vi "BRig_Host__Loop_Consumer_RunState__typeTrial__subtypeSelResult_parse__v3.vi"(0 "input_strCmd":string) -> (3 "output_selResult":bool, 4 "output_nTrial":u16, 6 "output_sSelection":u16, 8 "output_tSelection":u16, 10 "output_iReward_or_iError":u16, 12 "output_DAB_flipLR":u16, 13 "output_trig_l2":u16, 14 "output_trig_l1":u16, 15 "output_LorR":u16)   [LabVIEW 2014]
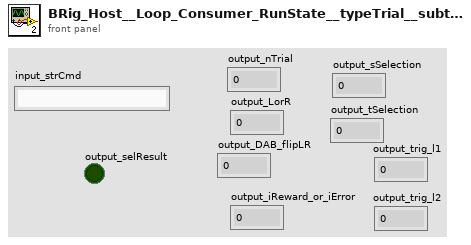
[diagram p1: front panel]
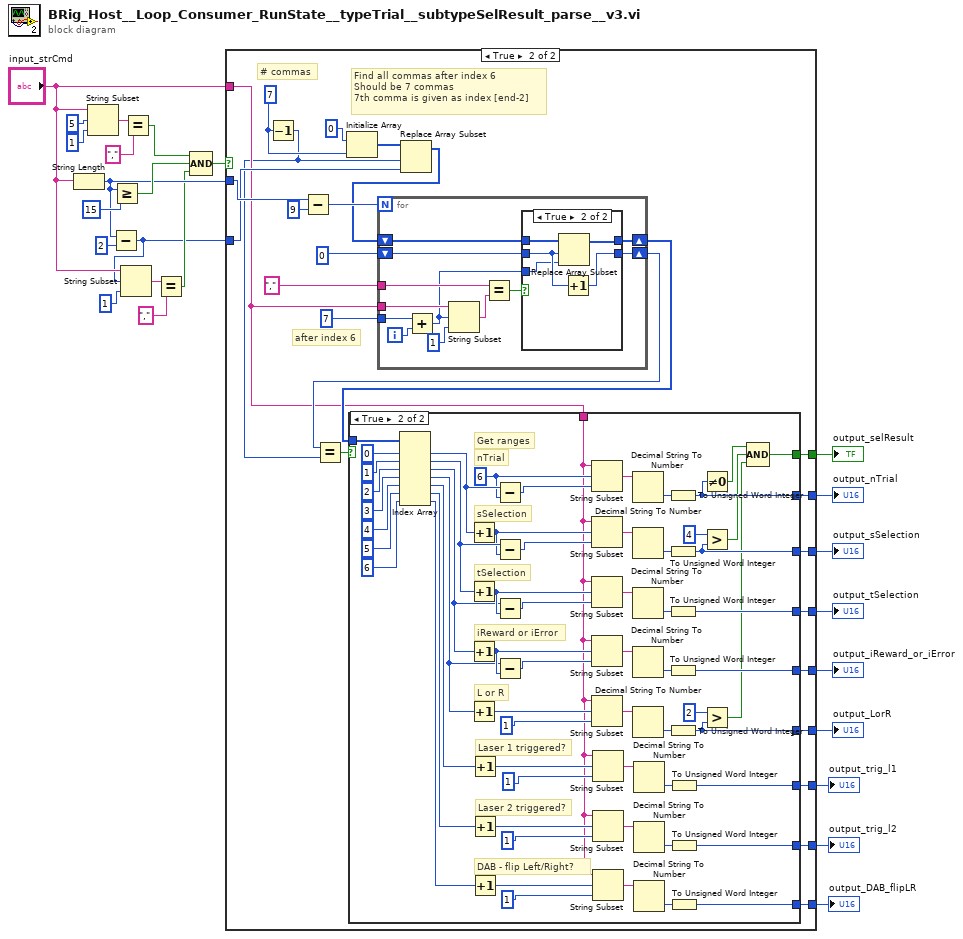
[diagram p0: block diagram]
diagram:
  n1 = String Length(string="input_strCmd") -> (length=w13:i32)
  n2 = String Subset(string="input_strCmd", offset (0)=5, length (rest)=1 ("offset (0)")) -> (substring=w23:string)
  n3 = Subtract(x=w13, y=2) -> (x-y=w10:i32)
  n4 = Greater Or Equal?(x=w13, y=15) -> (x >= y?=w20:bool)
  n5 = String Subset(string="input_strCmd", offset (0)=w10, length (rest)=1 ("offset (0)")) -> (substring=w15:string)
  n6 = Equal?(x=w23, y=",") -> (x = y?=w19:bool)
  n7 = Equal?(x=w15, y=",") -> (x = y?=w11:bool)
  n8 = Compound Arithmetic op=AND(w19, w20, w11) -> (w18:bool)
  n9 = case shown="True" w18 {
    tunnel: "input_strCmd" -> [_ w38]
    tunnel: w13 -> [_ w48]
    tunnel: w10 -> [_ w40]
    tunnel: [_ w36] -> w9
    tunnel: [_ w35] -> w8
    tunnel: [_ w34] -> w7
    tunnel: [_ w33] -> w6
    tunnel: [_ w32] -> w5
    tunnel: [_ w31] -> w4
    tunnel: [_ w28] -> w3
    tunnel: [_ w27] -> w2
    tunnel: [_ w26] -> w1
    frame False {
    }
    frame True {
      w30 = 7 ("dimension size")
      # "# commas"
      # "after index 6"
      # "Find all commas after index 6\nShould be 7 commas\n7th comma is given as index [end-2]"
      n10 = Decrement(x=w30) -> (x-1=w29:i32)
      n11 = Subtract(x=w48, y=9) -> (x-y=w47:i32)
      n12 = Initialize Array(0 ("element"), w30) -> (w42:i32[])
      n13 = Replace Array Subset(array=w42, new element=w40, index=w29) -> (w41:i32[])
      n14 = for {
        N: w47 -> [_]
        tunnel: w38 -> [w123]
        tunnel: "," ("y") -> [w121]
        tunnel: 7 ("element") -> [w119]
        shift-right: [w113] -> w43
        shift-left: 0 ("element") -> [w115]
        shift-right: [w114] -> w39
        shift-left: w41 -> [w116]
        i -> [w120]
        n15 = Add(x=w119, y=w120) -> (x+y=w117:i32)
        n16 = String Subset(string=w123, offset (0)=w117, length (rest)=1 ("offset (0)")) -> (substring=w122:string)
        n17 = Equal?(x=w121, y=w122) -> (x = y?=w118:bool)
        n18 = case shown="True" w118 {
          tunnel: w117 -> [_ w128]
          tunnel: w116 -> [w126 w131]
          tunnel: w115 -> [w125 w129]
          tunnel: [w126 w130] -> w114
          tunnel: [w125 w127] -> w113
          frame False {
          }
          frame True {
            n19 = Replace Array Subset(array=w131, new element=w128, index=w129) -> (w130:i32[])
            n20 = Increment(x=w129) -> (x+1=w127:i32)
          }
        }
      }
      n21 = Equal?(x=w43, y=w29) -> (x = y?=w37:bool)
      n22 = case shown="True" w37 {
        tunnel: w39 -> [_ w112]
        tunnel: w38 -> [_ w51]
        tunnel: [_ w81] -> w36
        tunnel: [_ w77] -> w35
        tunnel: [_ w80] -> w34
        tunnel: [_ w91] -> w33
        tunnel: [_ w90] -> w32
        tunnel: [_ w73] -> w31
        tunnel: [_ w60] -> w28
        tunnel: [_ w59] -> w27
        tunnel: [_ w52] -> w26
        frame False {
        }
        frame True {
          w88 = 6 ("y")
          # "DAB - flip Left/Right?"
          # "Laser 2 triggered?"
          # "Laser 1 triggered?"
          # "L or R"
          # "iReward or iError"
          # "tSelection"
          # "sSelection"
          # "nTrial"
          # "Get ranges"
          n23 = Index Array(array=w112, index #1=0 ("index"), index #2=1 ("index"), index #3=2 ("index"), index #4=3 ("index"), index #5=4 ("index"), index #6=5 ("index"), index #7=6 ("index")) -> (element #1=w89:i32, element #2=w87:i32, element #3=w82:i32, element #4=w84:i32, element #5=w63:i32, element #6=w62:i32, element #7=w53:i32)
          n24 = Increment(x=w89) -> (x+1=w86:i32)
          n25 = Increment(x=w87) -> (x+1=w83:i32)
          n26 = Increment(x=w82) -> (x+1=w85:i32)
          n27 = Increment(x=w84) -> (x+1=w103:i32)
          n28 = Increment(x=w63) -> (x+1=w64:i32)
          n29 = Increment(x=w62) -> (x+1=w70:i32)
          n30 = Increment(x=w53) -> (x+1=w57:i32)
          n31 = Subtract(x=w89, y=w88) -> (x-y=w107:i32)
          n32 = Subtract(x=w87, y=w86) -> (x-y=w106:i32)
          n33 = Subtract(x=w82, y=w83) -> (x-y=w105:i32)
          n34 = Subtract(x=w84, y=w85) -> (x-y=w104:i32)
          n35 = String Subset(string=w51, offset (0)=w88, length (rest)=w107) -> (substring=w101:string)
          n36 = String Subset(string=w51, offset (0)=w86, length (rest)=w106) -> (substring=w100:string)
          n37 = String Subset(string=w51, offset (0)=w83, length (rest)=w105) -> (substring=w99:string)
          n38 = String Subset(string=w51, offset (0)=w85, length (rest)=w104) -> (substring=w98:string)
          n39 = String Subset(string=w51, offset (0)=w103, length (rest)=1 ("y")) -> (substring=w97:string)
          n40 = String Subset(string=w51, offset (0)=w64, length (rest)=1 ("y")) -> (substring=w68:string)
          n41 = String Subset(string=w51, offset (0)=w70, length (rest)=1 ("y")) -> (substring=w67:string)
          n42 = String Subset(string=w51, offset (0)=w57, length (rest)=1 ("y")) -> (substring=w55:string)
          n43 = Decimal String To Number(string=w101) -> (number=w96:i32)  [unwired: 2 in, 1 out]
          n44 = Decimal String To Number(string=w100) -> (number=w95:i32)  [unwired: 2 in, 1 out]
          n45 = Decimal String To Number(string=w99) -> (number=w94:i32)  [unwired: 2 in, 1 out]
          n46 = Decimal String To Number(string=w98) -> (number=w93:i32)  [unwired: 2 in, 1 out]
          n47 = Decimal String To Number(string=w97) -> (number=w92:i32)  [unwired: 2 in, 1 out]
          n48 = Decimal String To Number(string=w68) -> (number=w66:i32)  [unwired: 2 in, 1 out]
          n49 = Decimal String To Number(string=w67) -> (number=w65:i32)  [unwired: 2 in, 1 out]
          n50 = Decimal String To Number(string=w55) -> (number=w54:i32)  [unwired: 2 in, 1 out]
          n51 = To Unsigned Word Integer(number=w96) -> (unsigned 16bit integer=w81:u16)
          n52 = To Unsigned Word Integer(number=w95) -> (unsigned 16bit integer=w80:u16)
          n53 = To Unsigned Word Integer(number=w94) -> (unsigned 16bit integer=w91:u16)
          n54 = To Unsigned Word Integer(number=w93) -> (unsigned 16bit integer=w90:u16)
          n55 = To Unsigned Word Integer(number=w92) -> (unsigned 16bit integer=w77:u16)
          n56 = To Unsigned Word Integer(number=w66) -> (unsigned 16bit integer=w60:u16)
          n57 = To Unsigned Word Integer(number=w65) -> (unsigned 16bit integer=w59:u16)
          n58 = To Unsigned Word Integer(number=w54) -> (unsigned 16bit integer=w52:u16)
          n59 = Not Equal To 0?(x=w81) -> (x != 0?=w74:bool)
          n60 = Greater?(x=u16 4, y=w80) -> (0:w75:bool)
          n61 = Greater?(x=u16 2, y=w77) -> (0:w76:bool)
          n62 = Compound Arithmetic op=AND(w74, w75, w76) -> (w73:bool)
        }
      }
    }
  }
  "output_nTrial" <- w9
  "output_LorR" <- w8
  "output_selResult" <- w4
  "output_sSelection" <- w7
  "output_tSelection" <- w6
  "output_iReward_or_iError" <- w5
  "output_trig_l1" <- w3
  "output_trig_l2" <- w2
  "output_DAB_flipLR" <- w1
